vi "Add.vi"(7 "startup?":bool=TRUE, 8 "error in (no error)":errorcluster, 10 "ProjectItem Refnum":refnum<vi>, 11 "EXE in":refnum<class "NI_AB_API_EXE.lvclass">) -> (0 "error out":errorcluster, 3 "EXE out":refnum<class "NI_AB_API_EXE.lvclass">)   [LabVIEW 2020, in "NI_AB_API_EXE.lvclass"]
uses:
  <vilib>/AppBuilder/AB_API/EXE/NI_AB_API_EXE.lvclass
  e:/builds/penguin/labview/branches/2020/dev/dist/vi.lib/AppBuilder/AB_API/Build/NI_AB_API_Build.lvclass
  <vilib>/AppBuilder/AB_Classes/EXE/AB_EXE.lvclass
  e:/builds/penguin/labview/branches/2020/dev/dist/vi.lib/AppBuilder/AB_Classes/Build/AB_Build.lvclass
  <vilib>/AppBuilder/AB_Classes/Build/AB_Build.lvclass
  <vilib>/AppBuilder/AB_Classes/Source/AB_Source.lvclass
  <vilib>/AppBuilder/AB_API/Build/NI_AB_API_Build.lvclass
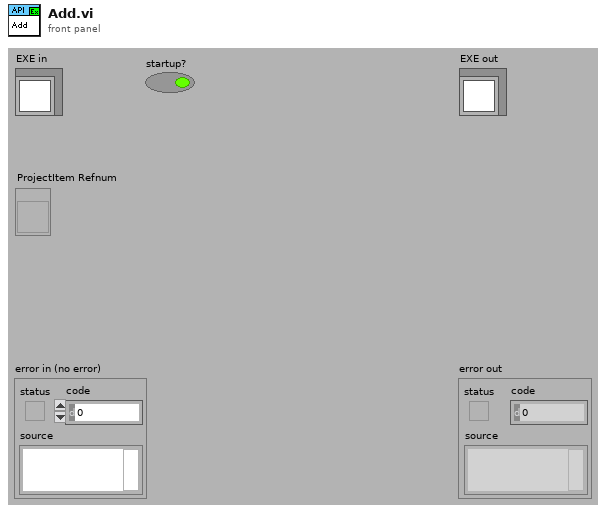
[diagram p1: front panel]
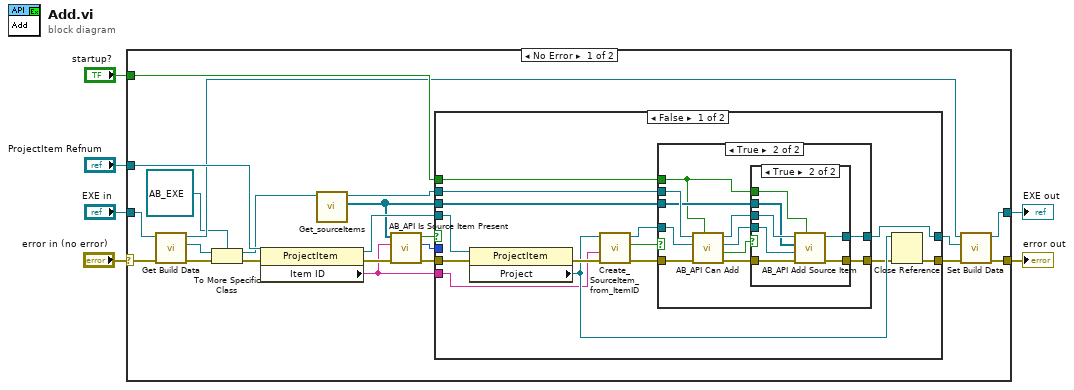
[diagram p0: block diagram]
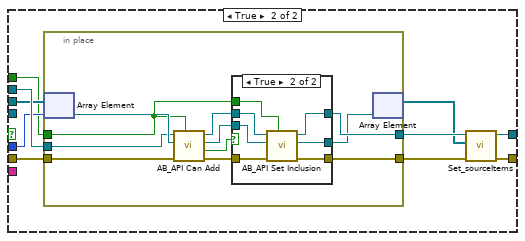
[diagram p4: hidden frame]
diagram:
  n1 = case shown="No Error" "error in (no error)" {
    selector: "error in (no error)" -> [w12 w97]
    tunnel: [w14 w97] -> w5
    tunnel: [w16 w96] -> w3
    tunnel: "EXE in" -> [w17 w96]
    tunnel: "ProjectItem Refnum" -> [w28 _]
    tunnel: "startup?" -> [w27 _]
    frame No Error {
      n2 = call <vilib>:"Get Build Data.vi"("error in (no error)"=w12, "NI_AB_API_Build in"=w17) -> ("error out"=w8:errorcluster, "AB_Build.lvclass"=w11:refnum<class "AB_Build.lvclass">, "NI_AB_API_Build out"=w18:refnum<class "NI_AB_API_EXE.lvclass">)  [unwired: 7 in]
      n3 = To More Specific Class(target class=refnum<class "AB_EXE.lvclass"> refnum ("AB_EXE.lvclass"), reference=w11, error in=w8) -> (specific class reference=w10:refnum<class "AB_EXE.lvclass">, error out=w7:errorcluster)
      n4 = property class="ProjectItem"(reference=w28, error in=w7) -> (reference out=w26:refnum<vi>, error out=w21:errorcluster, "Item ID"=w20:string)
      n5 = call <vilib>:"Get_sourceItems.vi"("Class in"=w10) -> ("sourceItems"=w25:refnum<class "AB_Source.lvclass">[], "Class out"=w24:refnum<class "AB_EXE.lvclass">)  [unwired: 1 in, 8 out]
      n6 = call <vilib>:"AB_API Is Source Item Present.vi"("error in"=w21, "item ID"=w20, "source items"=w25) -> ("error out"=w22:errorcluster, "index"=w19:i32, "source item present?"=w23:bool)  [unwired: 3 in, 3 out]
      n7 = case shown="False" w23 {
        tunnel: w26 -> [w42 _]
        tunnel: [w38 w68] -> w15
        tunnel: [w34 w71] -> w13
        tunnel: w22 -> [w33 w70]
        tunnel: w24 -> [w32 w69]
        tunnel: w20 -> [w31 _]
        tunnel: w25 -> [w30 w67]
        tunnel: w19 -> [_ w66]
        tunnel: w27 -> [w29 w65]
        frame False {
          n8 = property class="ProjectItem"(reference=w42, error in=w33) -> (error out=w41:errorcluster, "Project"=w36:refnum<vi>)  [unwired: 1 out]
          n9 = call <vilib>:"Create_SourceItem_from_ItemID.vi"("error in (no error)"=w41, "itemID"=w31, "Project Refnum"=w36) -> ("error out"=w39:errorcluster, "valid?"=w37:bool, "AB_Source out"=w40:refnum<class "AB_Source.lvclass">)  [unwired: 6 out]
          n10 = case shown="True" w37 {
            tunnel: w40 -> [_ w50]
            tunnel: w39 -> [w43 w48]
            tunnel: w32 -> [w44 w53]
            tunnel: [w44 w55] -> w38
            tunnel: [w43 w54] -> w35
            tunnel: w30 -> [_ w51]
            tunnel: w29 -> [_ w46]
            frame False {
            }
            frame True {
              n11 = call <vilib>:"AB_API Can Add.vi"("top tree? (true)"=w46, "error in (no error)"=w48, "AB_Source in"=w50, "Build in"=w53) -> ("error out"=w47:errorcluster, "can add?"=w45:bool, "AB_Source out"=w49:refnum<class "AB_Source.lvclass">, "Build out"=w52:refnum<class "AB_EXE.lvclass">)  [unwired: 4 in]
              n12 = case shown="True" w45 {
                tunnel: w52 -> [w57 w64]
                tunnel: [w57 w59] -> w55
                tunnel: [w56 w60] -> w54
                tunnel: w47 -> [w56 w63]
                tunnel: w49 -> [_ w61]
                tunnel: w51 -> [_ w62]
                tunnel: w46 -> [_ w58]
                frame False {
                }
                frame True {
                  n13 = call <vilib>:"AB_API Add Source Item.vi"("top tree? (true)"=w58, "error in"=w63, "Source in"=w61, "source items"=w62, "Build in"=w64) -> ("error out"=w60:errorcluster, "Build out"=w59:refnum<class "AB_EXE.lvclass">)  [unwired: 3 in, 2 out]
                }
              }
            }
          }
          n14 = Close Reference(reference=w36, error in (no error)=w35) -> (error out=w34:errorcluster)
        }
        frame True {
          n15 = in-place {
            in-place-border: [w85] -> w74
            in-place-border: w69 -> [w78]
            in-place-border: w70 -> [w82]
            in-place-border: [w84] -> w72
            in-place-border: w65 -> [w75]
            n16 = in-place-array #1(w67, w66) -> (w80:refnum<class "AB_Source.lvclass">)
            n17 = call <vilib>:"AB_API Can Add.vi"("top tree? (true)"=w75, "error in (no error)"=w82, "AB_Source in"=w80, "Build in"=w78) -> ("error out"=w81:errorcluster, "can add?"=w76:bool, "AB_Source out"=w79:refnum<class "AB_Source.lvclass">, "Build out"=w77:refnum<class "AB_EXE.lvclass">)  [unwired: 4 in]
            n18 = case shown="True" w76 {
              tunnel: [w86 w90] -> w84
              tunnel: [w88 w95] -> w85
              tunnel: w77 -> [w88 w93]
              tunnel: w79 -> [w87 w92]
              tunnel: w81 -> [w86 w91]
              tunnel: [w87 w94] -> w83
              tunnel: w75 -> [_ w89]
              frame False {
              }
              frame True {
                n19 = call <vilib>:"AB_API Set Inclusion.vi"("top tree? (true)"=w89, "error in (no error)"=w91, "Source in"=w92, "Build in"=w93) -> ("error out"=w90:errorcluster, "AB_Source_VI out"=w94:refnum<class "AB_Source.lvclass">, "AB_Build out"=w95:refnum<class "AB_EXE.lvclass">)  [unwired: 5 in]
              }
            }
            n20 = in-place-array #1(w83) -> (w73:refnum<class "AB_Source.lvclass">[])  [unwired: 1 out]
          }
          n21 = call <vilib>:"Set_sourceItems.vi"("error in (no error)"=w72, "sourceItems"=w73, "Class in"=w74) -> ("error out"=w71:errorcluster, "Class out"=w68:refnum<class "AB_EXE.lvclass">)  [unwired: 7 out]
        }
      }
      n22 = call <vilib>:"Set Build Data.vi"("error in (no error)"=w13, "AB_Build.lvclass"=w15, "NI_AB_API_Build in"=w18) -> ("error out"=w14:errorcluster, "NI_AB_API_Build out"=w16:refnum<class "NI_AB_API_EXE.lvclass">)  [unwired: 7 in]
    }
    frame Error {
    }
  }
  "error out" <- w5
  "EXE out" <- w3
